vi "Read_TurbiIN.vi"(0 "Refnum in":refnum<k21>, 1 "#Datos":i32=10 caption="Datos a Tomar" min=2 max=2500 step=1, 5 "error in (no error)":errorcluster) -> (14 "Datos":dbl[][](array[numeric]), 17 "size(s)":i32[](array[numeric]), 19 "error out":errorcluster)   [LabVIEW 2013]
uses:
  <vilib>/DAQmx/read.llb/DAQmx Read (Analog 2D DBL NChan NSamp).vi
  <vilib>/DAQmx/miscellaneous.llb/DAQmx Fill In Error Info.vi
panel:
  # "Columnas"
  # "Filas"
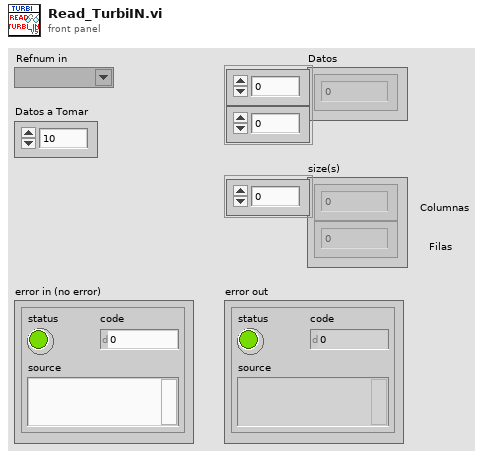
[diagram p1: front panel]
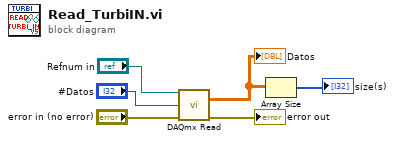
[diagram p0: block diagram]
diagram:
  n1 = call-poly <vilib>:"DAQmx Read.vi"("task/channels in"="Refnum in", "number of samples per channel"="#Datos", "error in"="error in (no error)") -> ("data"=w3:dbl[][], "error out"=→"error out":errorcluster)  [unwired: 10 in, 1 out]
  "Datos" <- w3
  n2 = Array Size(array=w3) -> (size(s)=→"size(s)":i32[])
